vi "main.vi"   [LabVIEW 2017, in "Demo.lvclass"]
uses:
  Demo.lvclass
  YoutuberDownloader Class/YoutuberDownloader.lvclass
  YoutubeCacheProxy Class/YoutubeCacheProxy.lvclass
  C:/Users/fflores/Documents/LabVIEW-Open-Projects/LabIVEW OOP Design Patterns/Proxy Pattern/ThirdPartyYoutubeLib Class/ThirdPartyYoutubeLib.lvclass
  ConsoleOut/Print Options.ctl
  ThirdPartyYoutubeClass Class/ThirdPartyYoutubeClass.lvclass
  YoutuberDownloader Class/YoutuberDownloader.lvclass/YoutuberDownloader.ctl
  ThirdPartyYoutubeLib Class/ThirdPartyYoutubeLib.lvclass
types:
  T1 = typedef "Print Options.ctl" = enum16{"Create", "Get Reference", "Print", "Print Header", "Close"}
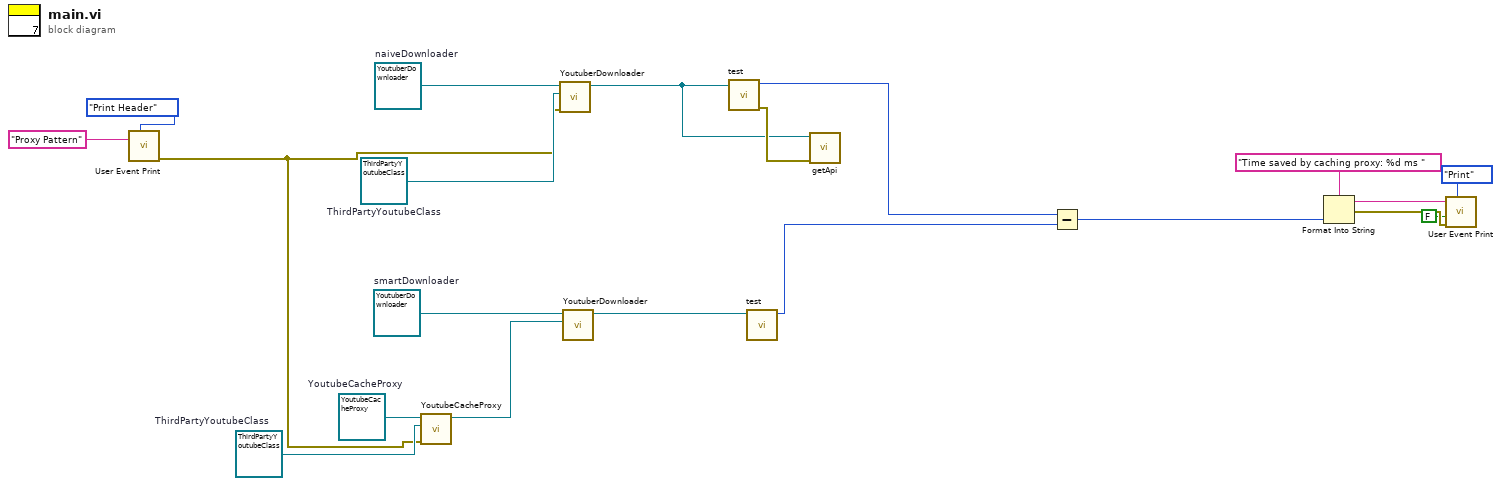
[diagram p0: block diagram]
diagram:
  w5 = refnum<class "ThirdPartyYoutubeClass.lvclass"> refnum  # ThirdPartyYoutubeClass
  w16 = refnum<class "ThirdPartyYoutubeClass.lvclass"> refnum  # ThirdPartyYoutubeClass
  w18 = refnum<class "YoutubeCacheProxy.lvclass"> refnum  # YoutubeCacheProxy
  w19 = refnum<class "YoutuberDownloader.lvclass"> refnum  # smartDownloader
  w20 = refnum<class "YoutuberDownloader.lvclass"> refnum  # naiveDownloader
  n1 = call "User Event Print.vi"("Options"=Print_Options."Print Header", "String to Print"="Proxy Pattern") -> ("error out"=w3:errorcluster)  [unwired: 8 in, 1 out]
  n2 = call "YoutubeCacheProxy.vi"("error in (no error)"=w3, "ThirdPartyYoutubeLib.lvclass"=w5, "YoutubeCacheProxy in"=w18) -> ("YoutubeCacheProxy out"=w17:refnum<class "YoutubeCacheProxy.lvclass">)  [unwired: 7 in, 1 out]
  n3 = call "YoutuberDownloader.vi"("error in (no error)"=w3, "ThirdPartyYoutubeLib.lvclass"=w16, "YoutuberDownloader in"=w20) -> ("YoutuberDownloader out"=w6:refnum<class "YoutuberDownloader.lvclass">)  [unwired: 7 in, 1 out]
  n4 = call "YoutuberDownloader.vi"("ThirdPartyYoutubeLib.lvclass"=w17, "YoutuberDownloader in"=w19) -> ("YoutuberDownloader out"=w15:refnum<class "YoutuberDownloader.lvclass">)  [unwired: 8 in, 1 out]
  n5 = call "test.vi"("YoutuberDownloader"=w6) -> ("error out"=w7:errorcluster, "estimatedTime"=w14:u32)  [unwired: 9 in]
  n6 = call "test.vi"("YoutuberDownloader"=w15) -> ("estimatedTime"=w13:u32)  [unwired: 9 in, 1 out]
  n7 = call "getApi.vi"("error in (no error)"=w7, "YoutuberDownloader in"=w6) -> ()  [unwired: 7 in, 3 out]
  n8 = Subtract(x=w14, y=w13) -> (x-y=w11:u32)
  n9 = Format Into String(format string="Time saved by caching proxy: %d ms ", w11) -> (resulting string=w10:string, error out=w9:errorcluster)  [unwired: 2 in]
  n10 = call "User Event Print.vi"("Options"=Print_Options."Print", "error in (no error)"=w9, "add EOL? (T)"=FALSE, "String to Print"=w10) -> ()  [unwired: 6 in, 2 out]
